vi "Write max queue size.vi"(8 "error in (no error)":errorcluster, 10 "max queue size":i32, 11 "bt_Send_Queue in":refnum<class "bt_Send_Queue.lvclass">) -> (0 "error out":errorcluster, 3 "bt_Send_Queue out":refnum<class "bt_Send_Queue.lvclass">)   [LabVIEW 2021, in "BT.lvlib" / "bt_Send_Queue.lvclass"]
uses:
  bt_Send_Queue.lvclass
  bt_Send_Queue.lvclass/bt_Send_Queue.ctl
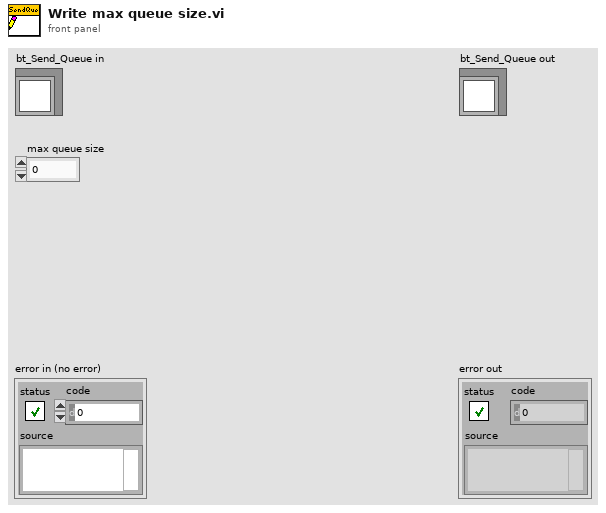
[diagram p1: front panel]
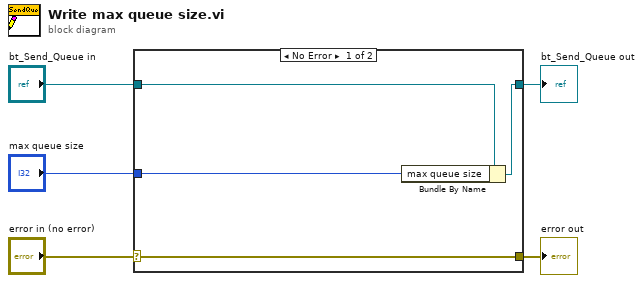
[diagram p0: block diagram]
diagram:
  n1 = case shown="No Error" "error in (no error)" {
    selector: "error in (no error)" -> [w9 w10]
    tunnel: [w9 w10] -> w4
    tunnel: [w7 w11] -> w2
    tunnel: "bt_Send_Queue in" -> [w8 w11]
    tunnel: "max queue size" -> [w6 _]
    frame No Error {
      n2 = Bundle By Name(cluster=w8, "max queue size"=w6) -> (w7:refnum<class "bt_Send_Queue.lvclass">)
    }
    frame Error {
    }
  }
  "error out" <- w4
  "bt_Send_Queue out" <- w2
